vi "Part 1.vi"(11 "Input":string="714892711431131262132720221453126624699325914653497873272491823531123510909339273820224452407894936892511248875491241226309223658524208482407275183819803893981238951393117621559881306698618296608681543653203748116999546983787150387751297422419423302719228339964412475926361848314117158155489366203640193571778983763559893452555799305618201784647864902896434223677019827554652620895433284524378618964266984994411654262114401369397065429922282240284651137140606858169661297332399986661123648223734045957885756837124716334270256968316689976235699897728581484794946740724336243413561355793014868146474971...") -> (3 "Output":i64)   [LabVIEW 2021]
uses:
  891bd29e-39a3-47c9-bc4b-203f6565d1c3.vi
  <userlib>/_OpenG.lib/string/string.llb/Convert EOLs (String)__ogtk.vi
  <vilib>/Comparison/Equal/Equal Functor/Equal Functor.lvclass
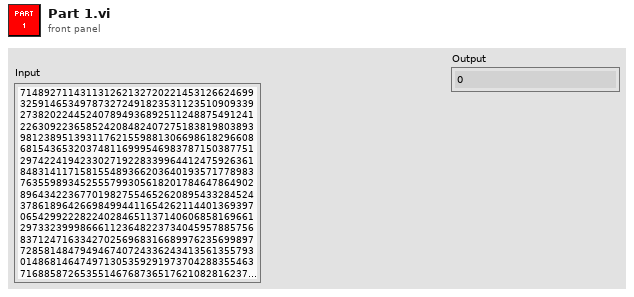
[diagram p1: front panel]
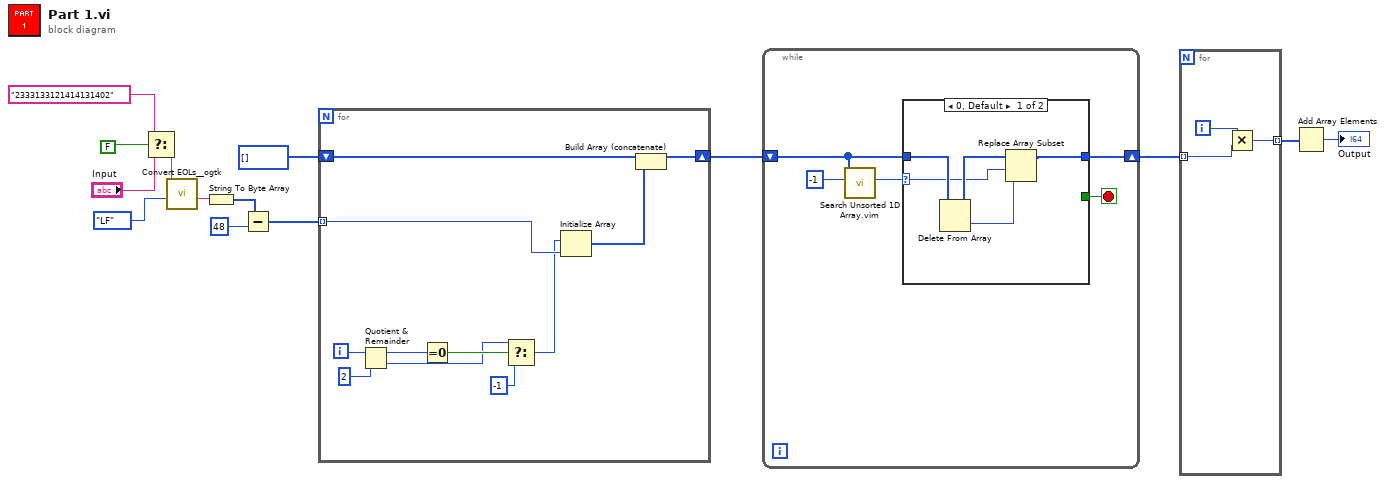
[diagram p0: block diagram]
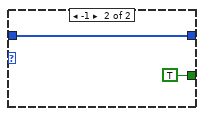
[diagram p2: hidden frame]
diagram:
  n1 = Select(t="2333133121414131402", s=FALSE, f="Input") -> (s? t:f=w6:string)
  n2 = call-poly <userlib>:"Convert EOLs__ogtk.vi"("Convert to:"=enum16{"CR", "LF", "CRLF"}."LF", "String in"=w6) -> ("String out"=w13:string)  [unwired: 9 in]
  n3 = String To Byte Array(string=w13) -> (unsigned byte array=w11:u8[])
  n4 = Subtract(x=w11, y=i64 48) -> (x-y=w10:i64[])
  n5 = for {
    tunnel: w10 -> [w19] mode=indexing
    shift-right: [w15] -> w4
    shift-left: i64[] [] -> [w16]
    i -> [w25]
    n6 = Quotient & Remainder(x=w25, y=2) -> (x-y*floor(x/y)=w23:i32, floor(x/y)=w21:i32)
    n7 = Equal To 0?(x=w23) -> (x = 0?=w22:bool)
    n8 = Select(t=w21, s=w22, f=-1) -> (s? t:f=w18:i32)
    n9 = Initialize Array(w18, w19) -> (w17:i32[])
    n10 = Build Array (concatenate)(w16, w17) -> (w15:i64[])
  }
  n11 = while {
    shift-right: [w26] -> w3
    shift-left: w4 -> [w27]
    stop <- w28 stop-if-true
    n12 = call "Search Unsorted 1D Array.vim"("element"=-1, "unsorted 1D array"=w27) -> ("index of element"=w29:i32)  [unwired: 9 in]
    n13 = case shown="0, Default" w29 {
      selector: w29 -> [w31 _]
      tunnel: [_ TRUE] -> w28
      tunnel: w27 -> [w33 w36]
      tunnel: [w35 w36] -> w26
      frame 0, Default {
        n14 = Delete From Array(array=w33) -> (deleted portion=w32:i64, array with subset deleted=w34:i64[])  [unwired: 2 in]
        n15 = Replace Array Subset(array=w34, new element=w32, index=w31) -> (w35:i64[])
      }
      frame -1 {
      }
    }
  }
  n16 = for {
    tunnel: w3 -> [w40] mode=indexing
    tunnel: [w38] -> w2 mode=indexing
    i -> [w39]
    n17 = Multiply(x=w39, y=w40) -> (x*y=w38:i64)
  }
  n18 = Add Array Elements(numeric array=w2) -> (sum=→"Output":i64)
